vi "T7 Read Cal Constants KAG.vi"(0 "IP Configuration":T1={"Connection ID In"=refnum, "Connection ID Out"=refnum, "Device IP"="192.168.126.147", "Port"=502}, 4 "Flash Write Registers":T5(array[cluster])=[{"Register Num"=61800, "Register Name"="INTERNAL_FLASH_KEY", "DataType"="UINT32", "Write Val"=1134709826.0}, {"Register Num"=61810, "Register Name"="INTERNAL_FLASH_READ_POINTER", "DataType"="UINT32", "Write Val"=3948544.0}] {"Write Val" format="%#.0f"}, 5 "Stream Configuration":T3={"Scan Rate (Hz)"=1000.0, "Samples Per Packet"=512, "Resolution Index"=0, "Buffer Size (bytes)"=32768, "NumScans"=1500, "Read Timeout (ms)"=5000, "Scan Table"=[{"Channel"=0, "BipGain"=0, "Input Config"="Single-Ended"}, {"Channel"=1, "BipGain"=0, "Input Config"="Single-Ended"}, {"Channel"=2, "BipGain"=0, "Input Config"="Single-Ended"}, {"Channel"=3, "BipGain"=0, "Input Config"="Single-Ended"}]} {"Samples Per Packet" max=512 step=1; "Buffer Size (bytes)" max=32768 step=1; "Resolution Index" max=8 step=1; "Scan Rate (Hz)" max=100000; "Scan Table"."BipGain" items=["x1", "x10", "x100", "x1000"]; "Scan Table"."Channel" step=1}, 6 "Flash Read Registers":T5(array[cluster])=[{"Register Num"=61812, "Register Name"="INTERNAL_FLASH_READ", "DataType"="UINT32", "Write Val"=0.0}], 7 "Secondary Stream Configurations":T2={"Settling Delay (*5 us)"=0.0, "Clock Source"=0, "Auto Target"=1} {"Auto Target" max=255 step=1; "Clock Source" max=2 step=2; "Settling Delay (*5 us)" min=0 max=5000 step=1}, 11 "error in":errorcluster) -> (8 "Calibration Constants":T6(array[cluster]) {"PSlope" format="%#.13f"; "NSlope" format="%#.13f"; "AvgSlope" format="%#.13f"; "Center" format="%#.13f"; "Offset" format="%#.13f"}, 15 "error out":errorcluster)   [LabVIEW 2015]
doc: "Write Stream Configuration LabJack Registers via MODBUS. There are a set of registers which comprise the stream configuration registers, and these are written with control values for Scan Rate, NumScans, Resolution, etc. Also, the Scan Table is used to build a Scan List of Stream Configuration Registers which point to streamable AI Channels."
uses:
  T7 Stream Config KAG.ctl
  T7 Secondary Configs KAG.ctl
  T7 IP Config KAG.ctl
  T7Examples/MODBUS/T7MOD_Write_UINT16_Register.vi
  T7Examples/MODBUS/T7MOD_Write_UINT32_Register.vi
  T7Examples/MODBUS/T7MOD_Write_FLOAT32_Register.vi
  T7Examples/MODBUS/T7MOD_Read_UINT16_Register.vi
  T7Examples/MODBUS/T7MOD_Read_FLOAT32_Register.vi
  T7 Stream Globals KAG.vi
panel:
  in  "Tab Control":T4(tab)=enum."Flash Data"
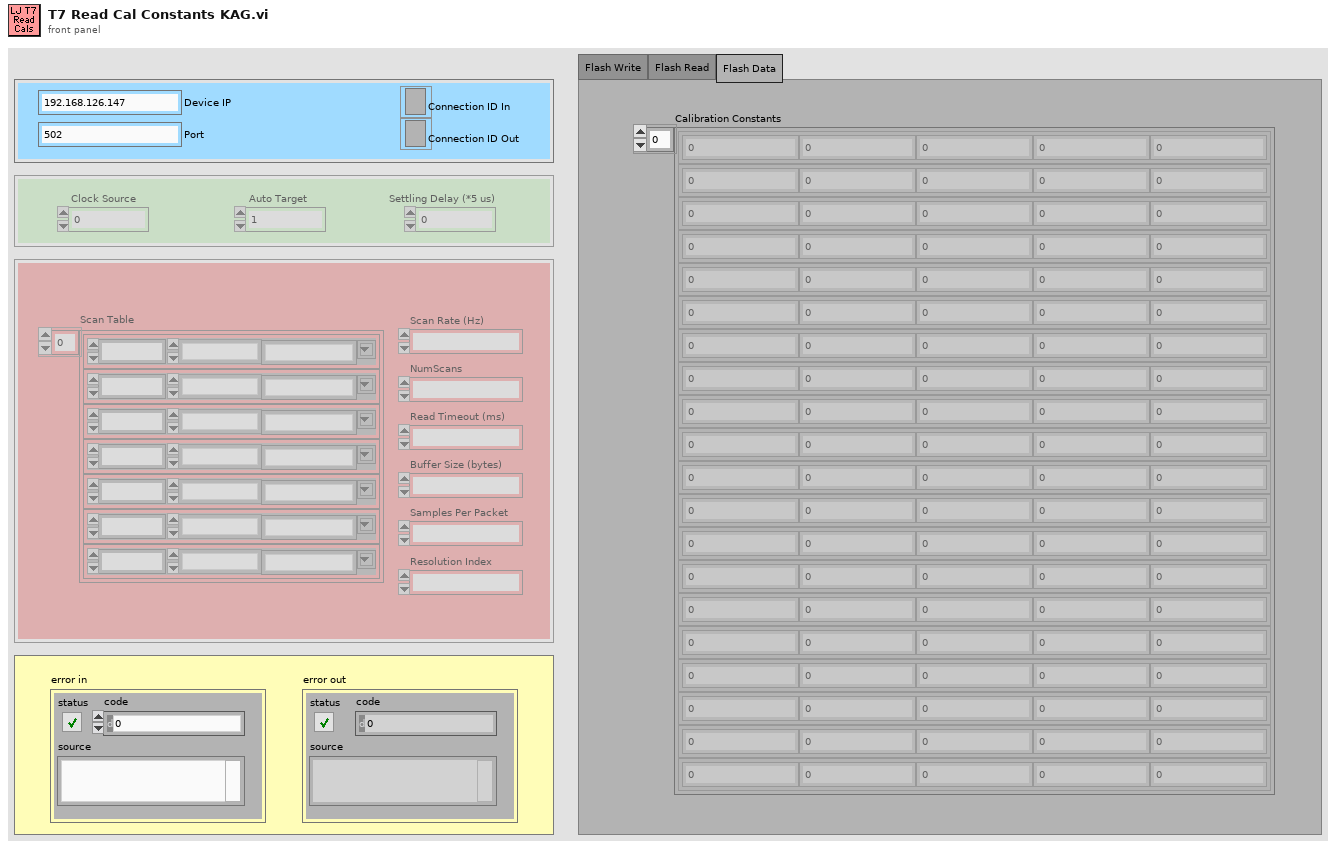
[diagram p1: front panel]
types:
  T1 = typedef "T7 IP Config KAG.ctl" = cluster{"Connection ID In":refnum<k5>, "Connection ID Out":refnum<k5>, "Device IP":string, "Port":i32}
  T2 = typedef "T7 Secondary Configs KAG.ctl" = cluster{"Settling Delay (*5 us)":sgl, "Clock Source":u32, "Auto Target":u32}
  T3 = typedef "T7 Stream Config KAG.ctl" = cluster{"Scan Rate (Hz)":sgl, "Samples Per Packet":u32, "Resolution Index":u32, "Buffer Size (bytes)":u32, "NumScans":u32, "Read Timeout (ms)":u32, "Scan Table":cluster{"Channel":u32, "BipGain":u32, "Input Config":string}[]}
  T4 = enum32{"Flash Write", "Flash Read", "Flash Data"}
  T5 = cluster{"Register Num":i32, "Register Name":string, "DataType":string, "Write Val":dbl}[]
  T6 = cluster{"PSlope":dbl, "NSlope":dbl, "AvgSlope":dbl, "Center":dbl, "Offset":dbl}[]
  T7 = cluster{"Register Num":i32, "Register Name":string, "DataType":string, "Write Val":dbl}
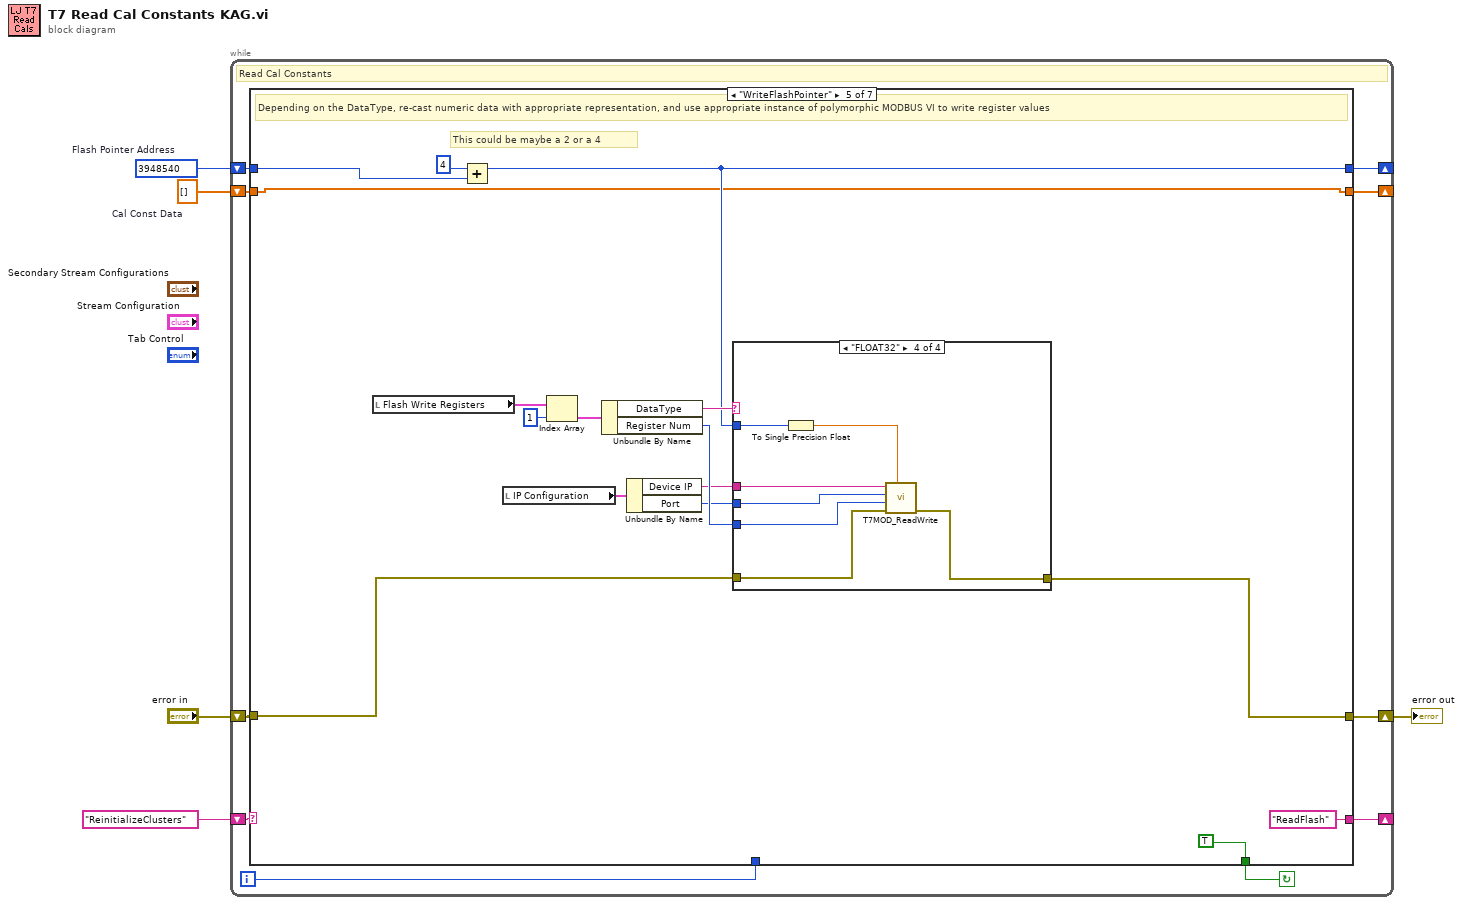
[diagram p0: block diagram]
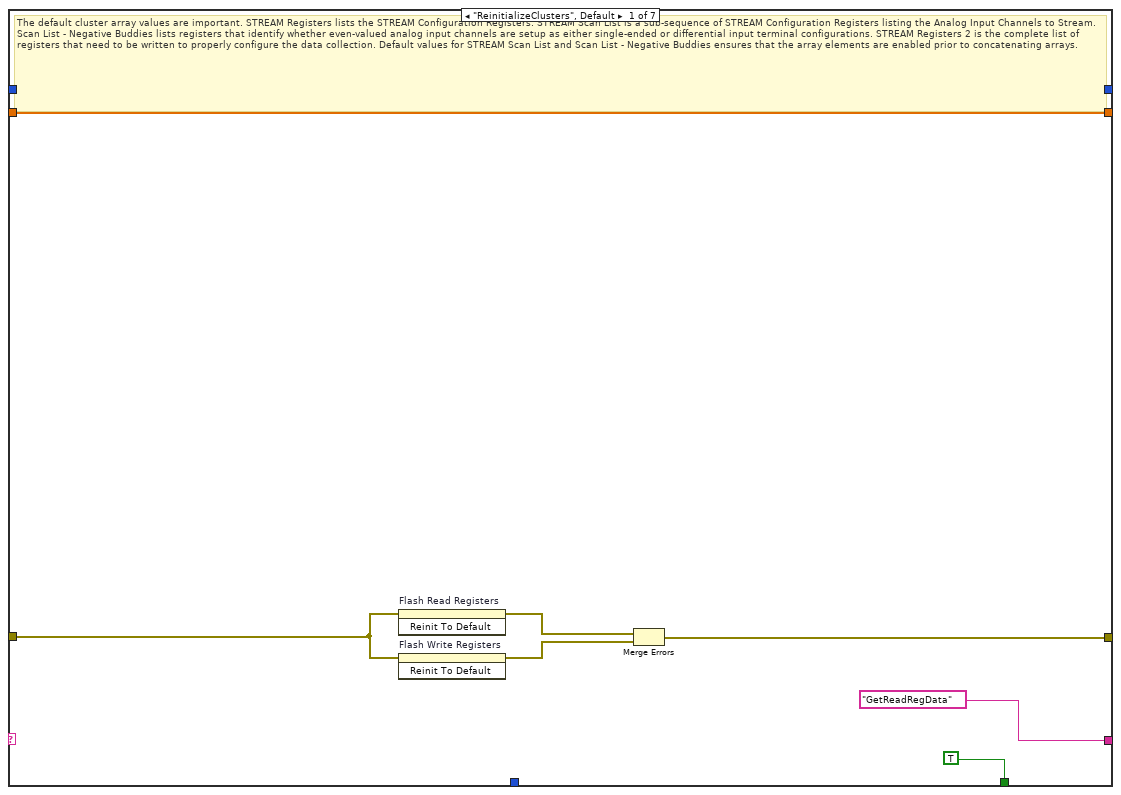
[diagram p2: hidden frame]
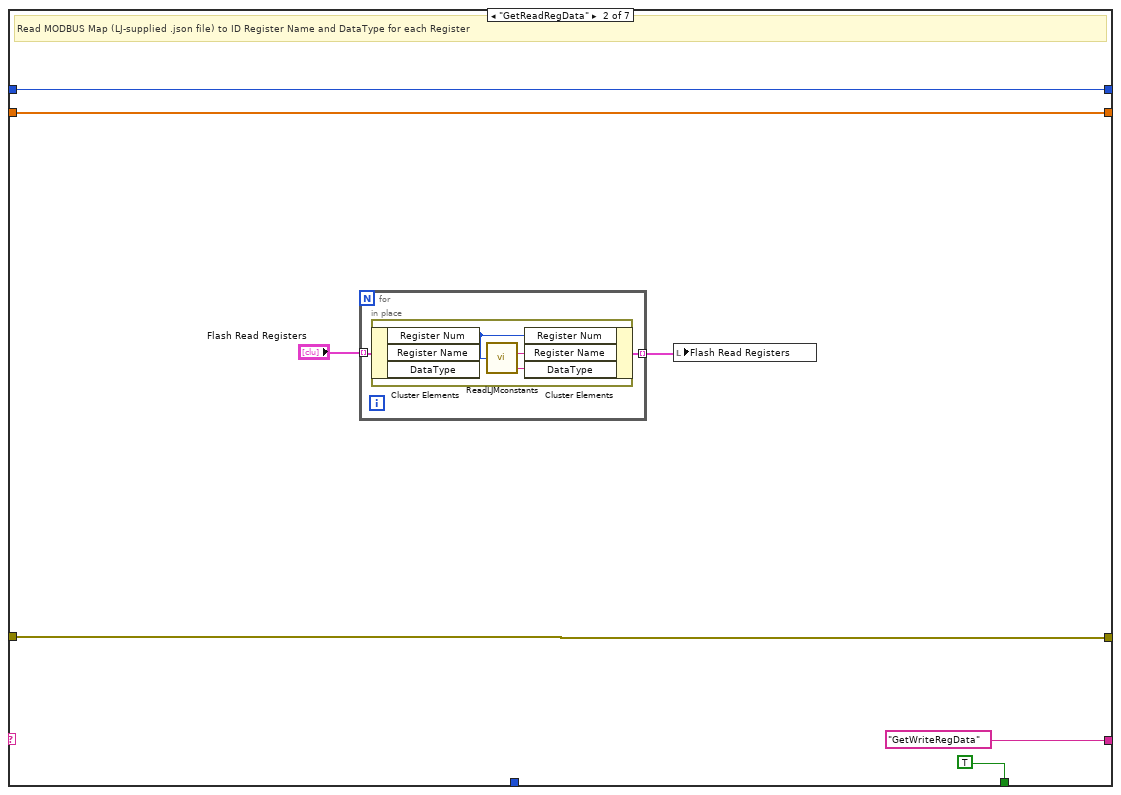
[diagram p3: hidden frame]
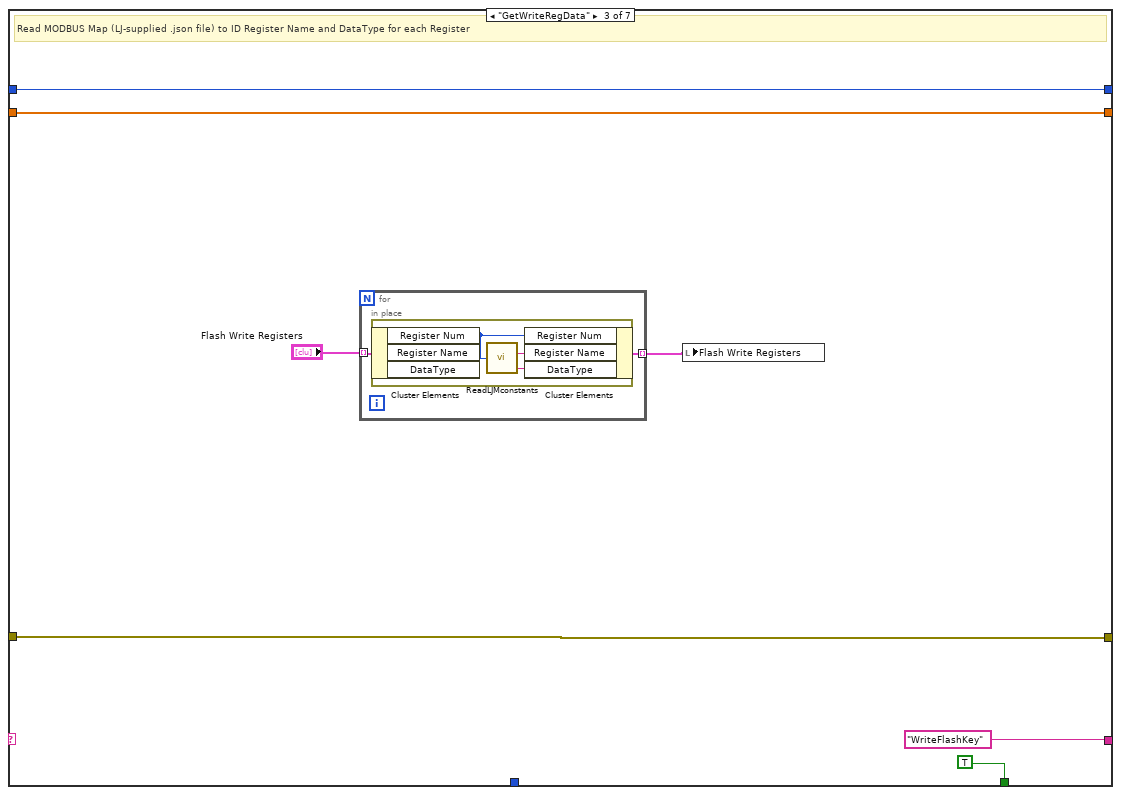
[diagram p4: hidden frame]
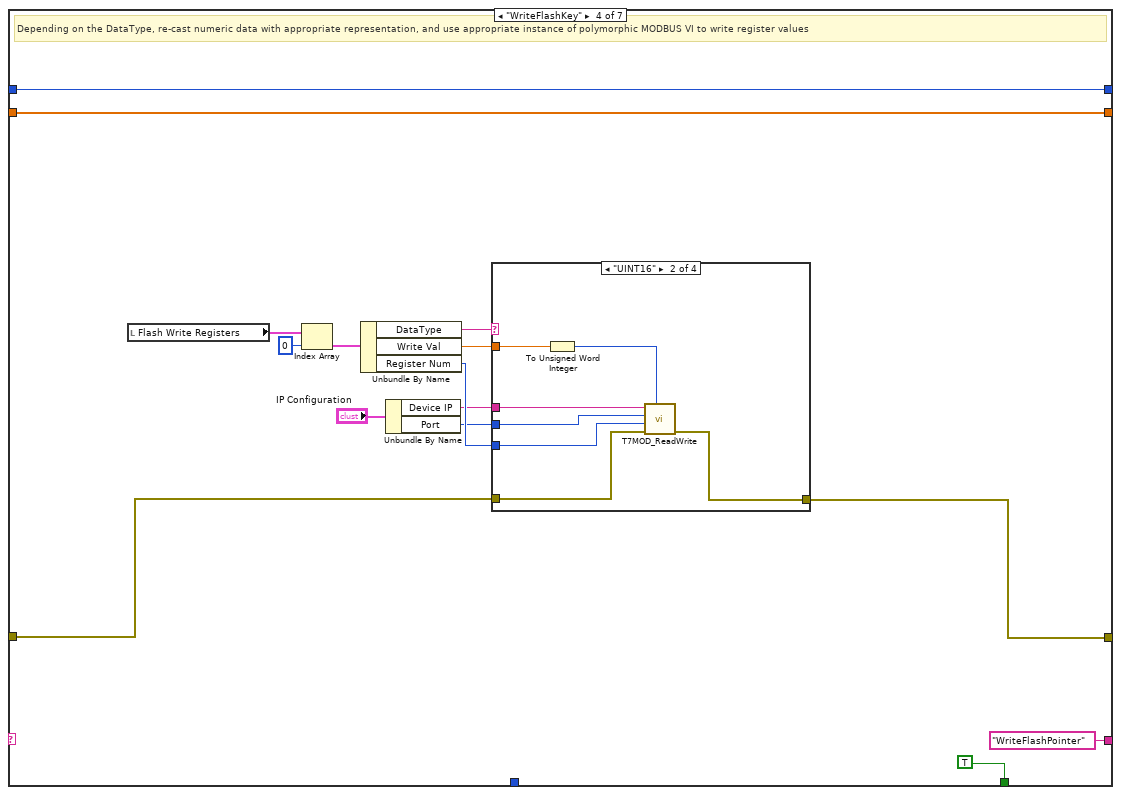
[diagram p5: hidden frame]
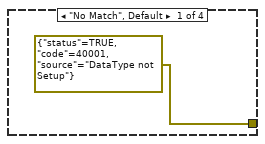
[diagram p6: hidden frame]
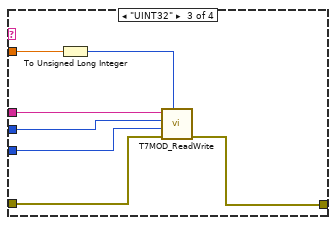
[diagram p7: hidden frame]
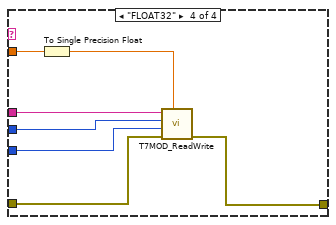
[diagram p8: hidden frame]
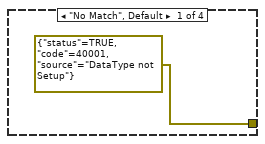
[diagram p9: hidden frame]
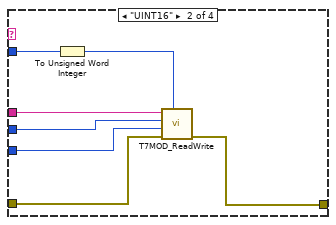
[diagram p10: hidden frame]
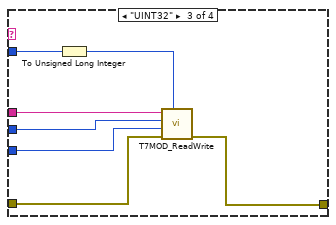
[diagram p11: hidden frame]
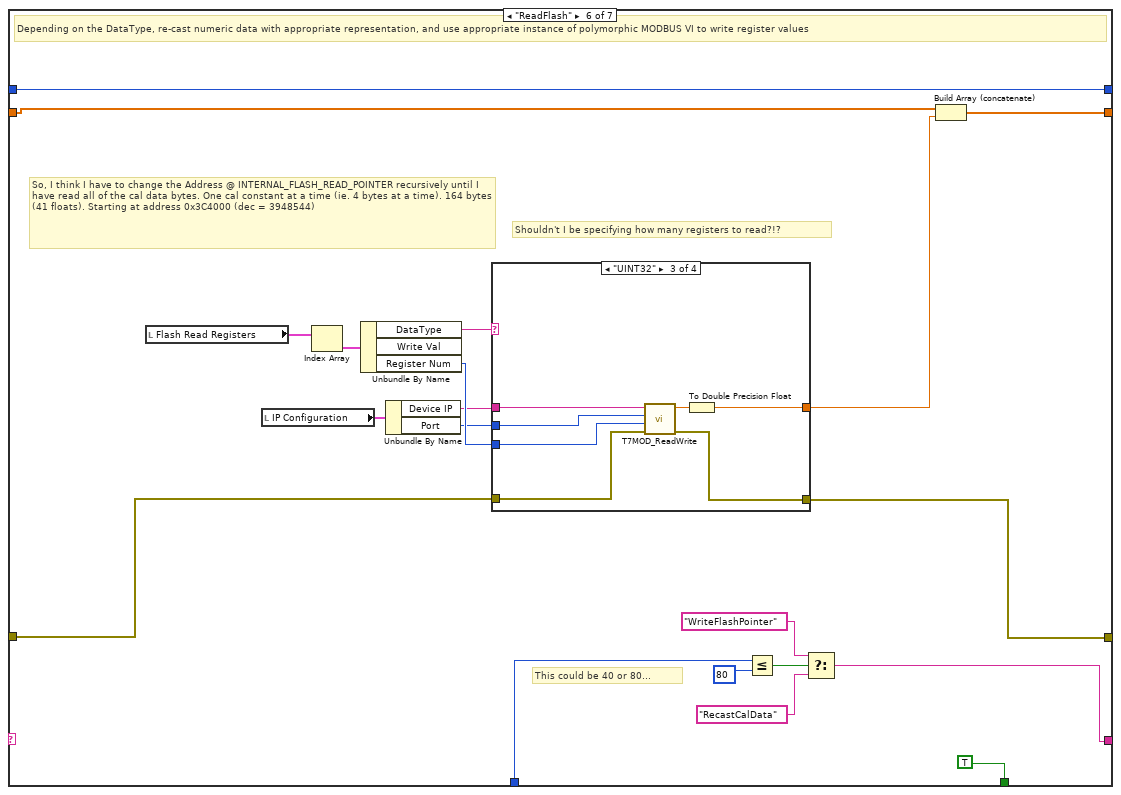
[diagram p12: hidden frame]
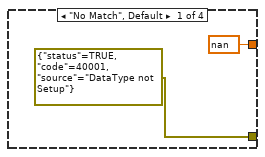
[diagram p13: hidden frame]
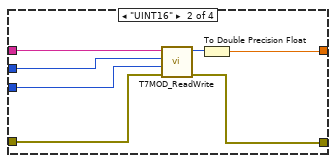
[diagram p14: hidden frame]
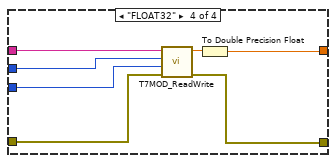
[diagram p15: hidden frame]
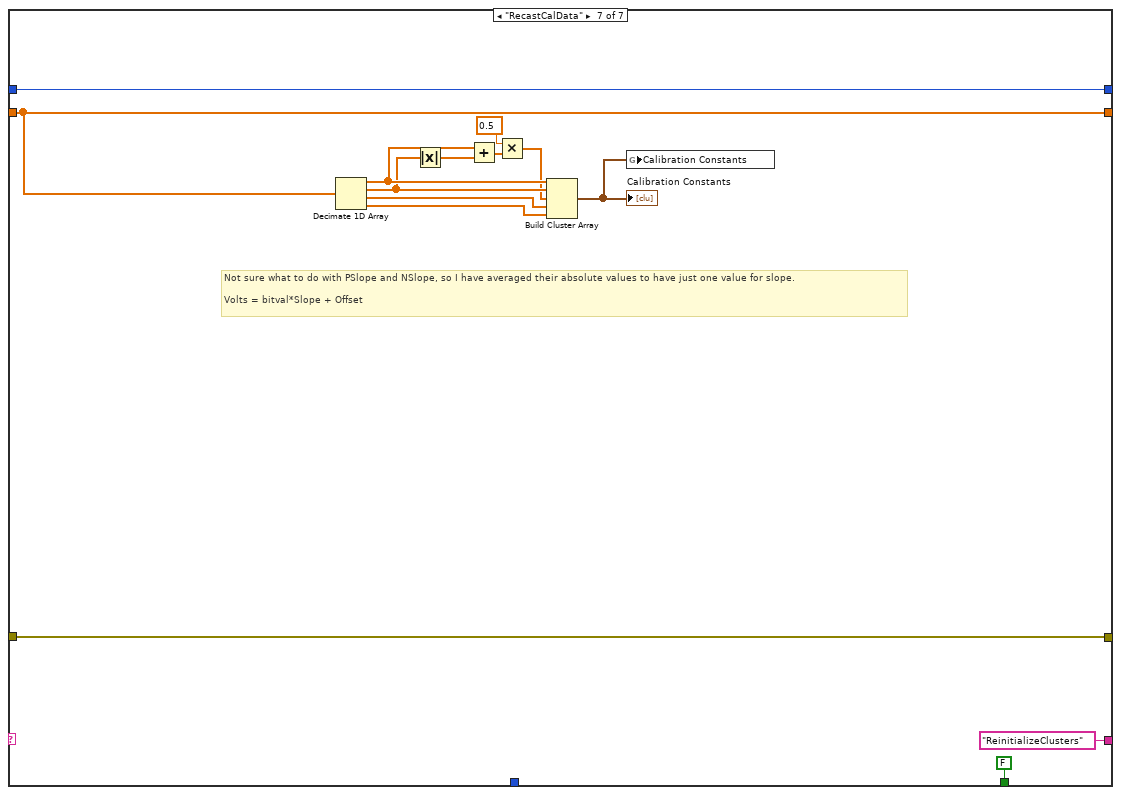
[diagram p16: hidden frame]
diagram:
  w1 = dbl[] []  # Cal Const Data
  w2 = u32 3948540  # Flash Pointer Address
  n1 = while {
    shift-right: [w13] -> _
    shift-left: "ReinitializeClusters" -> [w15]
    shift-right: [w11] -> w3
    shift-left: "error in" -> [w12]
    shift-right: [w10] -> _
    shift-left: w2 -> [w9]
    shift-right: [w7] -> _
    shift-left: w1 -> [w6]
    i -> [w8]
    stop <- w14 continue-if-true
    # "Read Cal Constants"
    n2 = case shown="\"WriteFlashPointer\"" w15 {
      tunnel: [TRUE TRUE TRUE TRUE TRUE TRUE FALSE] -> w14
      tunnel: ["GetReadRegData" "GetWriteRegData" "WriteFlashKey" "WriteFlashPointer" "ReadFlash" w126 "ReinitializeClusters"] -> w13
      tunnel: w12 -> [w21 w27 w39 w61 w99 w141 w175]
      tunnel: [w19 w27 w39 w60 w98 w140 w175] -> w11
      tunnel: [w17 w26 w38 w52 w91 w139 w178] -> w10
      tunnel: w9 -> [w17 w26 w38 w52 w88 w139 w178]
      tunnel: w8 -> [_ _ _ _ _ w131 _]
      tunnel: [w16 w25 w37 w51 w90 w134 w177] -> w7
      tunnel: w6 -> [w16 w25 w37 w51 w90 w133 w177]
      frame "ReinitializeClusters", Default {
        # "The default cluster array values are important. STREAM Registers lists the STREAM Configuration Registers. STREAM Scan List is a sub-sequence of STREAM Configuration Registers listing the Analog Input Channels to Stream. Scan List - Negative Buddies lists registers that identify whether even-valued analog input channels are setup as either single-ended or differential input terminal configurations. STREAM Registers 2 is the complete list of registers that need to be written to properly configure the data collection. Default values for STREAM Scan List and Scan List - Negative Buddies ensures that the array elements are enabled prior to concatenating arrays."
        n3 = invoke on="Flash Read Registers" class="Arr (strict)" method="Reinit To Default"(error in=w21) -> (error out=w20:errorcluster)  [unwired: 2 in, 2 out]
        n4 = invoke on="Flash Write Registers" class="Arr (strict)" method="Reinit To Default"(error in=w21) -> (error out=w18:errorcluster)  [unwired: 2 in, 2 out]
        n5 = Merge Errors(w20, w18) -> (w19:errorcluster)
      }
      frame "GetReadRegData" {
        # "Read MODBUS Map (LJ-supplied .json file) to ID Register Name and DataType for each Register"
        n6 = for {
          tunnel: "Flash Read Registers" -> [w32] mode=indexing
          tunnel: [w31] -> w28 mode=indexing
          n7 = in-place {
            n8 = in-place-cluster #1(w32) -> ("Register Num"=w33:i32)  [unwired: 2 out]
            n9 = call "ReadLJMconstants.vi"("Selected Register"=w33) -> ("Register Name"=w35:string, "Data Type"=w34:string)  [unwired: 1 out]
            n10 = in-place-cluster #1("Register Num"=w33, "Register Name"=w35, "DataType"=w34) -> (w31:T7)
          }
        }
        n11 = local write "Flash Read Registers"(w28) -> ()
      }
      frame "GetWriteRegData" {
        # "Read MODBUS Map (LJ-supplied .json file) to ID Register Name and DataType for each Register"
        n12 = for {
          tunnel: "Flash Write Registers" -> [w44] mode=indexing
          tunnel: [w43] -> w40 mode=indexing
          n13 = in-place {
            n14 = in-place-cluster #2(w44) -> ("Register Num"=w45:i32)  [unwired: 2 out]
            n15 = call "ReadLJMconstants.vi"("Selected Register"=w45) -> ("Register Name"=w47:string, "Data Type"=w46:string)  [unwired: 1 out]
            n16 = in-place-cluster #2("Register Num"=w45, "Register Name"=w47, "DataType"=w46) -> (w43:T7)
          }
        }
        n17 = local write "Flash Write Registers"(w40) -> ()
      }
      frame "WriteFlashKey" {
        # "Depending on the DataType, re-cast numeric data with appropriate representation, and use appropriate instance of polymorphic MODBUS VI to write register values"
        n18 = local read "Flash Write Registers"() -> (w55:T5)
        n19 = Index Array(array=w55, index=0) -> (element=w53:T7)
        n20 = Unbundle By Name(w53) -> ("DataType"=w58:string, "Write Val"=w57:dbl, "Register Num"=w56:i32)
        n21 = Unbundle By Name("IP Configuration") -> ("Device IP"=w49:string, "Port"=w48:i32)
        n22 = case shown="\"UINT16\"" w58 {
          tunnel: w57 -> [_ w70 w77 w84]
          tunnel: w56 -> [_ w69 w76 w83]
          tunnel: w61 -> [_ w68 w75 w82]
          tunnel: [errorcluster {"status"=TRUE, "code"=40001, "source"="DataType not Setup"} ("error constant") w67 w74 w81] -> w60
          tunnel: w49 -> [_ w66 w73 w80]
          tunnel: w48 -> [_ w65 w72 w79]
          frame "No Match", Default {
          }
          frame "UINT16" {
            n23 = To Unsigned Word Integer(number=w70) -> (unsigned 16bit integer=w64:u16)
            n24 = call-poly "T7MOD_ReadWrite.vi"("UINT16 to Write"=w64, "error in"=w68, "LabJack UINT16 Register"=w69, "Remote Port"=w65, "Remote IP Address"=w66) -> ("error out"=w67:errorcluster)  [unwired: 5 in, 1 out]
          }
          frame "UINT32" {
            n25 = To Unsigned Long Integer(number=w77) -> (unsigned 32bit integer=w71:u32)
            n26 = call-poly "T7MOD_ReadWrite.vi"("UINT32 to Write"=w71, "error in"=w75, "LabJack UINT32 Register"=w76, "Remote Port"=w72, "Remote IP Address"=w73) -> ("error out"=w74:errorcluster)  [unwired: 5 in, 1 out]
          }
          frame "FLOAT32" {
            n27 = To Single Precision Float(number=w84) -> (single precision float=w78:sgl)
            n28 = call-poly "T7MOD_ReadWrite.vi"("FLOAT32 to Write"=w78, "error in"=w82, "LabJack FLOAT32 Register"=w83, "Remote Port"=w79, "Remote IP Address"=w80) -> ("error out"=w81:errorcluster)  [unwired: 5 in, 1 out]
          }
        }
      }
      frame "WriteFlashPointer" {
        # "This could be maybe a 2 or a 4"
        # "Depending on the DataType, re-cast numeric data with appropriate representation, and use appropriate instance of polymorphic MODBUS VI to write register values"
        n29 = local read "Flash Write Registers"() -> (w95:T5)
        n30 = Add(x=u32 4 ("y"), y=w88) -> (x+y=w91:u32)
        n31 = local read "IP Configuration"() -> (w87:T1)
        n32 = Index Array(array=w95, index=1) -> (element=w93:T7)
        n33 = Unbundle By Name(w93) -> ("DataType"=w96:string, "Register Num"=w92:i32)
        n34 = Unbundle By Name(w87) -> ("Device IP"=w86:string, "Port"=w85:i32)
        n35 = case shown="\"FLOAT32\"" w96 {
          tunnel: w91 -> [_ w108 w115 w122]
          tunnel: w92 -> [_ w107 w114 w121]
          tunnel: w99 -> [_ w106 w113 w120]
          tunnel: [errorcluster {"status"=TRUE, "code"=40001, "source"="DataType not Setup"} ("error constant") w105 w112 w119] -> w98
          tunnel: w86 -> [_ w104 w111 w118]
          tunnel: w85 -> [_ w103 w110 w117]
          frame "No Match", Default {
          }
          frame "UINT16" {
            n36 = To Unsigned Word Integer(number=w108) -> (unsigned 16bit integer=w102:u16)
            n37 = call-poly "T7MOD_ReadWrite.vi"("UINT16 to Write"=w102, "error in"=w106, "LabJack UINT16 Register"=w107, "Remote Port"=w103, "Remote IP Address"=w104) -> ("error out"=w105:errorcluster)  [unwired: 5 in, 1 out]
          }
          frame "UINT32" {
            n38 = To Unsigned Long Integer(number=w115) -> (unsigned 32bit integer=w109:u32)
            n39 = call-poly "T7MOD_ReadWrite.vi"("UINT32 to Write"=w109, "error in"=w113, "LabJack UINT32 Register"=w114, "Remote Port"=w110, "Remote IP Address"=w111) -> ("error out"=w112:errorcluster)  [unwired: 5 in, 1 out]
          }
          frame "FLOAT32" {
            n40 = To Single Precision Float(number=w122) -> (single precision float=w116:sgl)
            n41 = call-poly "T7MOD_ReadWrite.vi"("FLOAT32 to Write"=w116, "error in"=w120, "LabJack FLOAT32 Register"=w121, "Remote Port"=w117, "Remote IP Address"=w118) -> ("error out"=w119:errorcluster)  [unwired: 5 in, 1 out]
          }
        }
      }
      frame "ReadFlash" {
        # "This could be 40 or 80..."
        # "Shouldn't I be specifying how many registers to read?!?"
        # "So, I think I have to change the Address @ INTERNAL_FLASH_READ_POINTER recursively until I have read all of the cal data bytes. One cal constant at a time (ie. 4 bytes at a time). 164 bytes (41 floats). Starting at address 0x3C4000 (dec = 3948544)"
        # "Depending on the DataType, re-cast numeric data with appropriate representation, and use appropriate instance of polymorphic MODBUS VI to write register values"
        n42 = local read "Flash Read Registers"() -> (w136:T5)
        n43 = local read "IP Configuration"() -> (w125:T1)
        n44 = Index Array(array=w136) -> (element=w135:T7)  [unwired: 1 in]
        n45 = Unbundle By Name(w135) -> ("DataType"=w138:string, "Register Num"=w137:i32)  [unwired: 1 out]
        n46 = Unbundle By Name(w125) -> ("Device IP"=w124:string, "Port"=w123:i32)
        n47 = case shown="\"UINT32\"" w138 {
          tunnel: w137 -> [_ w151 w158 w165]
          tunnel: w141 -> [_ w150 w157 w164]
          tunnel: [errorcluster {"status"=TRUE, "code"=40001, "source"="DataType not Setup"} ("error constant") w149 w156 w163] -> w140
          tunnel: w124 -> [_ w148 w155 w162]
          tunnel: w123 -> [_ w147 w154 w161]
          tunnel: [nan w145 w152 w159] -> w132
          frame "No Match", Default {
          }
          frame "UINT16" {
            n48 = call-poly "T7MOD_ReadWrite.vi"("error in"=w150, "LabJack UINT16 Register"=w151, "Remote Port"=w147, "Remote IP Address"=w148) -> ("error out"=w149:errorcluster, "Read UINT16"=w146:u16)  [unwired: 4 in, 2 out]
            n49 = To Double Precision Float(number=w146) -> (double precision float=w145:dbl)
          }
          frame "UINT32" {
            n50 = call-poly "T7MOD_ReadWrite.vi"("error in"=w157, "LabJack FLOAT32 Register"=w158, "Remote Port"=w154, "Remote IP Address"=w155) -> ("error out"=w156:errorcluster, "Read FLOAT32"=w153:sgl)  [unwired: 4 in, 2 out]
            n51 = To Double Precision Float(number=w153) -> (double precision float=w152:dbl)
          }
          frame "FLOAT32" {
            n52 = call-poly "T7MOD_ReadWrite.vi"("error in"=w164, "LabJack FLOAT32 Register"=w165, "Remote Port"=w161, "Remote IP Address"=w162) -> ("error out"=w163:errorcluster, "Read FLOAT32"=w160:sgl)  [unwired: 4 in, 2 out]
            n53 = To Double Precision Float(number=w160) -> (double precision float=w159:dbl)
          }
        }
        n54 = Less Or Equal?(x=w131, y=80) -> (x <= y?=w129:bool)
        n55 = Select(t="WriteFlashPointer", s=w129, f="RecastCalData") -> (s? t:f=w126:string)
        n56 = Build Array (concatenate)(w133, w132) -> (w134:dbl[])
      }
      frame "RecastCalData" {
        # "Not sure what to do with PSlope and NSlope, so I have averaged their absolute values to have just one value for slope.\n\nVolts = bitval*Slope + Offset"
        n57 = Decimate 1D Array(w177) -> (w174:dbl[], w173:dbl[], w169:dbl[], w168:dbl[])
        n58 = Absolute Value(x=w173) -> (abs(x)=w167:dbl[])
        n59 = Add(x=w174, y=w167) -> (x+y=w172:dbl[])
        n60 = Multiply(x=0.5, y=w172) -> (x*y=w170:dbl[])
        n61 = Build Cluster Array(w174, w173, w170, w169, w168) -> (w166:cluster{dbl, dbl, dbl, dbl, dbl}[])
        "Calibration Constants" <- w166
        n62 = global write "T7 Stream Globals KAG.vi" "Calibration Constants"(w166) -> ()
      }
    }
  }
  "error out" <- w3
